vi "Motion Sensor + security.vi"() -> ()   [LabVIEW 2011]
uses:
  <vilib>/LabVIEW Interface for Arduino/Type Defs/Board Type.ctl
  <vilib>/LabVIEW Interface for Arduino/LabVIEW Interface for Arduino.lvlib
panel:
  out "error out":errorcluster
  in  "error in":errorcluster
  out "Door Lock":bool
  in  "stop":bool
  out "Voltage":dbl(knob) scale=0.0..5.0
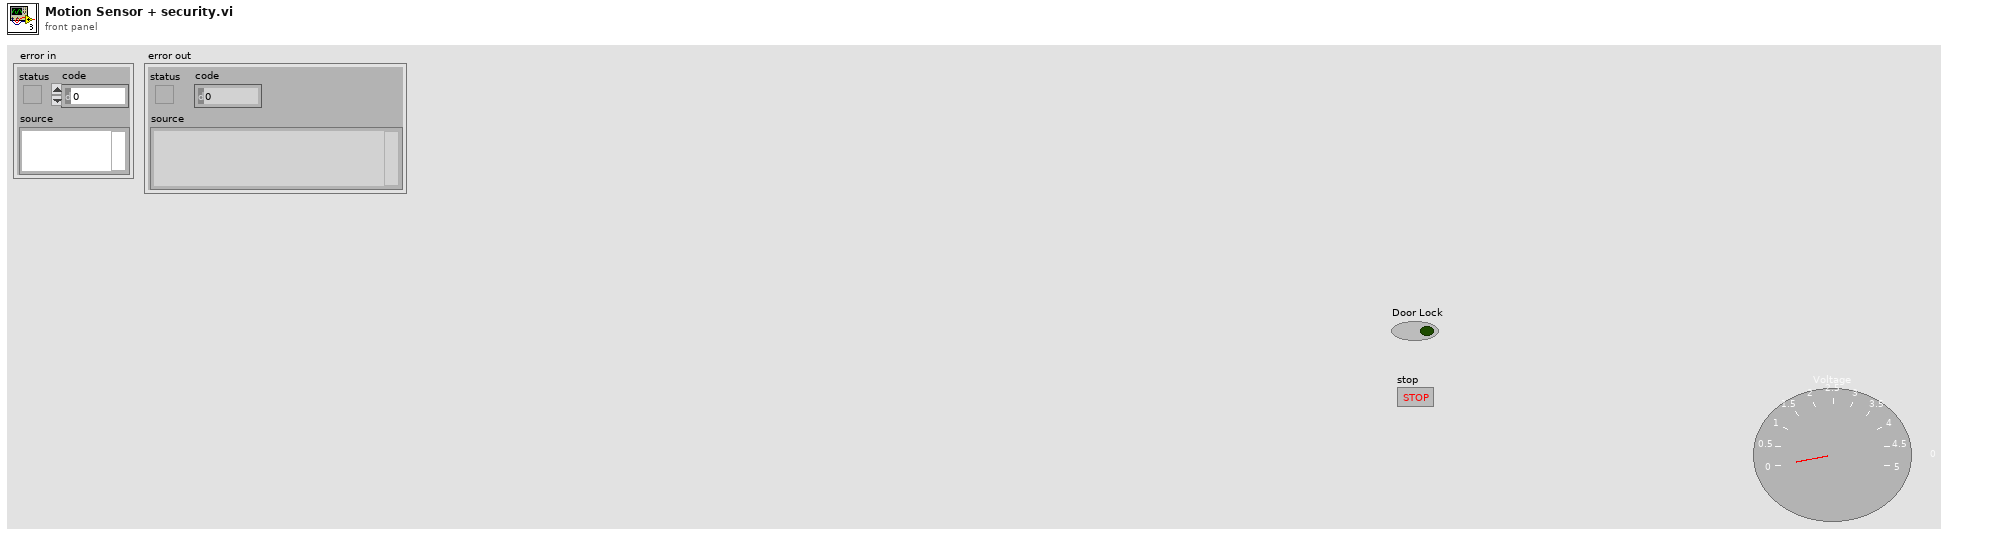
[diagram p1: front panel]
types:
  T1 = typedef "LabVIEW Interface for Arduino.lvlib/Board Type.ctl" = enum16{"Uno", "Dimuelanove w/Atmega 328", "Mega 2560"}
  T2 = typedef "LabVIEW Interface for Arduino.lvlib/Arduino Resource.ctl" = cluster{"VISA resource":refnum<visa-resource-name>, "Board Type":T1, "Connection Type":enum8{"USB / Serial"}, "Bytes Per Packet (15)":u8}
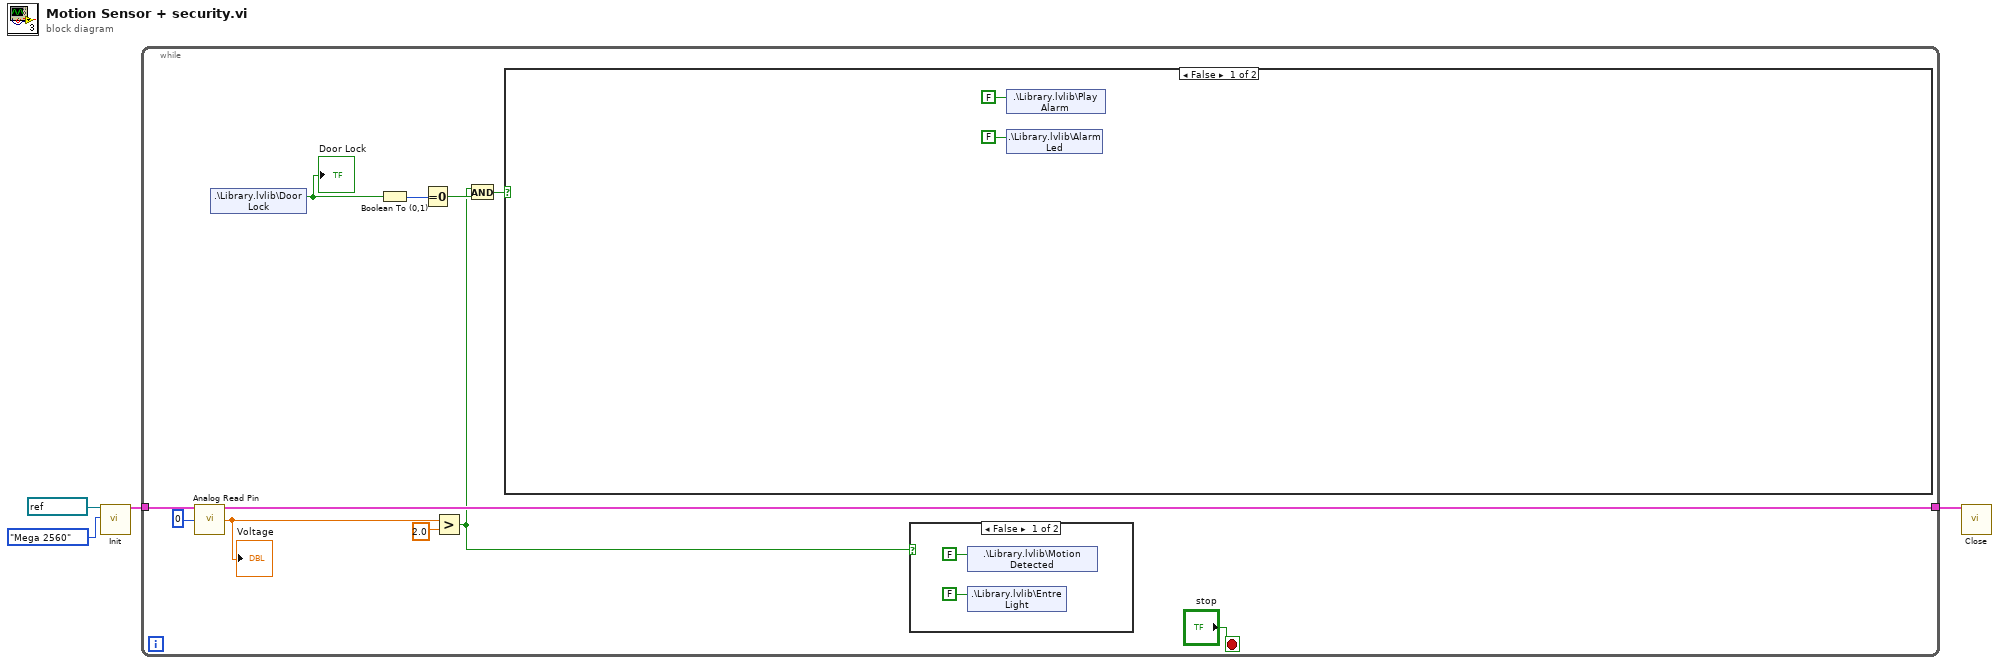
[diagram p0: block diagram]
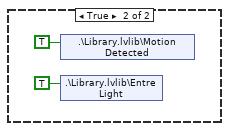
[diagram p2: hidden frame]
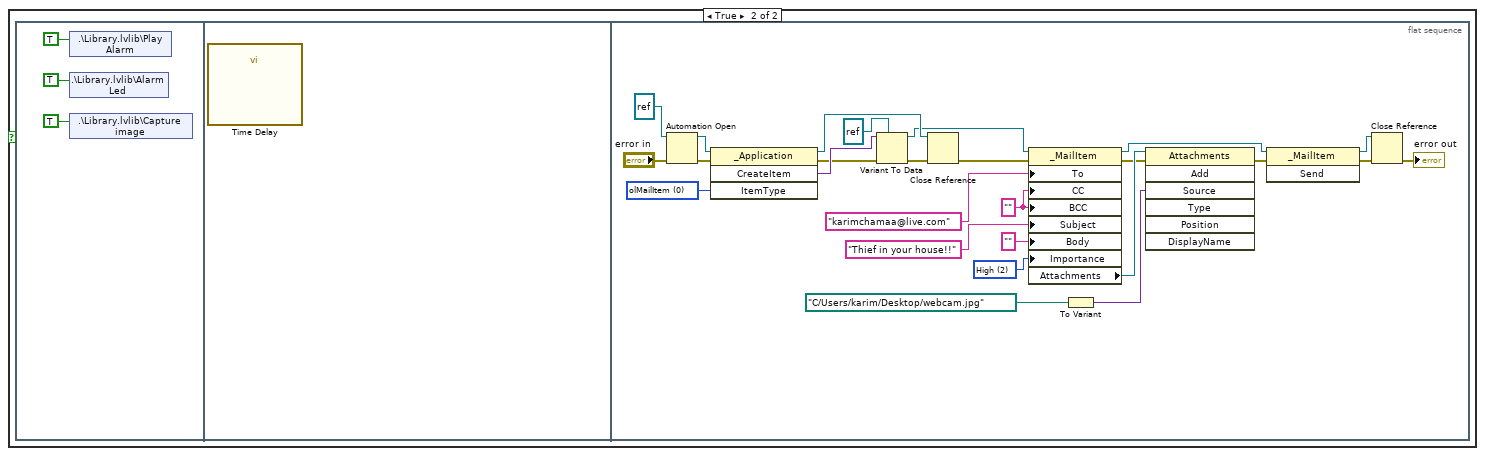
[diagram p3: hidden frame]
diagram:
  n1 = call <vilib>:"Init.vi"("VISA resource"=refnum<visa-resource-name> "COM4", "Board Type (Uno)"=Board_Type."Mega 2560") -> ("Arduino Resource"=w4:T2)  [unwired: 16 in, 1 out]
  n2 = while {
    tunnel: w4 -> [w14]
    tunnel: [w12] -> w3
    stop <- "stop" stop-if-true
    n3 = call <vilib>:"Analog Read Pin.vi"("Arduino Resource"=w14, "Analog Input Pin (0)"=u8 0) -> ("Arduino Resource"=w12:T2, "Voltage"=w11:dbl)  [unwired: 11 in, 1 out]
    "Voltage" <- w11
    n4 = shared-variable ".\\Library.lvlib\\Door Lock"() -> (w6:bool)  [unwired: 1 in, 1 out]
    "Door Lock" <- w6
    n5 = Boolean To (0,1)(Boolean=w6) -> (0, 1=w9:i16)
    n6 = Equal To 0?(x=w9) -> (x = 0?=w8:bool)
    n7 = Greater?(x=w11, y=2.0) -> (0:w5:bool)
    n8 = And(x=w5, y=w8) -> (x .and. y?=w7:bool)
    n9 = case shown="False" w7 {
      frame False {
        n10 = shared-variable ".\\Library.lvlib\\Play Alarm"(FALSE ("Play Alarm")) -> ()  [unwired: 1 in, 1 out]
        n11 = shared-variable ".\\Library.lvlib\\Alarm Led"(FALSE ("Capture image")) -> ()  [unwired: 1 in, 1 out]
      }
      frame True {
        n12 = flat-sequence {
          frame #0 {
            n13 = shared-variable ".\\Library.lvlib\\Play Alarm"(TRUE ("Play Alarm")) -> ()  [unwired: 1 in, 1 out]
            n14 = shared-variable ".\\Library.lvlib\\Alarm Led"(TRUE ("Capture image")) -> ()  [unwired: 1 in, 1 out]
            n15 = shared-variable ".\\Library.lvlib\\Capture image"(TRUE ("Capture image")) -> ()  [unwired: 1 in, 1 out]
          }
          frame #1 {
            n16 = call "Time Delay"() -> ()  [unwired: 11 in, 1 out]
          }
          frame #2 {
            w28 = "" ("CC")
            w29 = 2 items=["Low", "Normal", "High"] ("Importance")
            w47 = 0 items=["olMailItem", "olAppointmentItem", "olContactItem", "olTaskItem", "olJournalItem", "olNoteItem", "olPostItem"] ("ItemType")
            n17 = Automation Open(error in (no error)="error in", Automation Refnum=refnum<k7> refnum ("Outlook._Application")) -> (Automation Refnum=w48:refnum<k7>, error out=w41:errorcluster)  [unwired: 2 in]
            n18 = invoke class="_Application" method="CreateItem"(reference=w48, error in=w41, "ItemType"=w47) -> (reference out=w44:refnum<k7>, error out=w39:errorcluster, "CreateItem"=w46:variant)  [unwired: 1 in, 1 out]
            n19 = Variant To Data(error in=w39, type=refnum<k7> refnum ("Outlook._MailItem"), Variant=w46) -> (data=w30:refnum<k7>, error out=w38:errorcluster)
            n20 = Close Reference(reference=w44, error in (no error)=w38) -> (error out=w37:errorcluster)
            n21 = property class="_MailItem"(reference=w30, error in=w37, "To"="karimchamaa@live.com", "CC"=w28, "BCC"=w28, "Subject"="Thief in your house!!", "Body"="" ("Message"), "Importance"=w29) -> (reference out=w31:refnum<k7>, error out=w34:errorcluster, "Attachments"=w35:refnum<k7>)
            n22 = To Variant(anything=path "C:/Users/karim/Desktop/webcam.jpg" ("Report Path")) -> (Variant=w33:variant)
            n23 = invoke class="Attachments" method="Add"(reference=w35, error in=w34, "Source"=w33) -> (error out=w32:errorcluster)  [unwired: 4 in, 6 out]
            n24 = invoke class="_MailItem" method="Send"(reference=w31, error in=w32) -> (reference out=w43:refnum<k7>, error out=w42:errorcluster)  [unwired: 1 in, 1 out]
            n25 = Close Reference(reference=w43, error in (no error)=w42) -> (error out=→"error out":errorcluster)
          }
        }
      }
    }
    n26 = case shown="False" w5 {
      frame False {
        n27 = shared-variable ".\\Library.lvlib\\Motion Detected"(FALSE ("Motion Detected")) -> ()  [unwired: 1 in, 1 out]
        n28 = shared-variable ".\\Library.lvlib\\Entre Light"(FALSE ("Entre Light")) -> ()  [unwired: 1 in, 1 out]
      }
      frame True {
        n29 = shared-variable ".\\Library.lvlib\\Motion Detected"(TRUE ("Motion Detected")) -> ()  [unwired: 1 in, 1 out]
        n30 = shared-variable ".\\Library.lvlib\\Entre Light"(TRUE ("Entre Light")) -> ()  [unwired: 1 in, 1 out]
      }
    }
  }
  n31 = call <vilib>:"Close.vi"("Arduino Resource"=w3) -> ()  [unwired: 14 in, 1 out]
